vi "RGB_merge.vi"(7 "offset and range":T1[](array[typedef]) {"offset" min=0.0 max=1.0 step=0.0010000000474974513 scale=0.0..1.0; "range" min=0.0 max=1.0 step=0.0010000000474974513 scale=0.0..1.0}, 8 "error in (no error)":errorcluster, 9 "colours":T2[](array[typedef]), 10 "images":refnum<class "Image.lvclass">[](array[class]), 11 "Image in":refnum<class "Image.lvclass">=refnum) -> (0 "error out":errorcluster, 3 "Image out":refnum<class "Image.lvclass">)   [LabVIEW 2010, in "Image.lvclass"]
uses:
  Image.lvclass
  colour_enum.ctl
  clusters/range_offset_cluster.ctl
  storage_mode.ctl
  ErrorController/ErrorController/class_data.vi
  <vilib>/vision/NI_Vision_Development_Module.lvlib
  ErrorController/ErrorController/ErrorController.lvclass
panel:
  # "Note: \nIf offset and range value is not provided or empty, the intrinsic range offset of each image is taken."
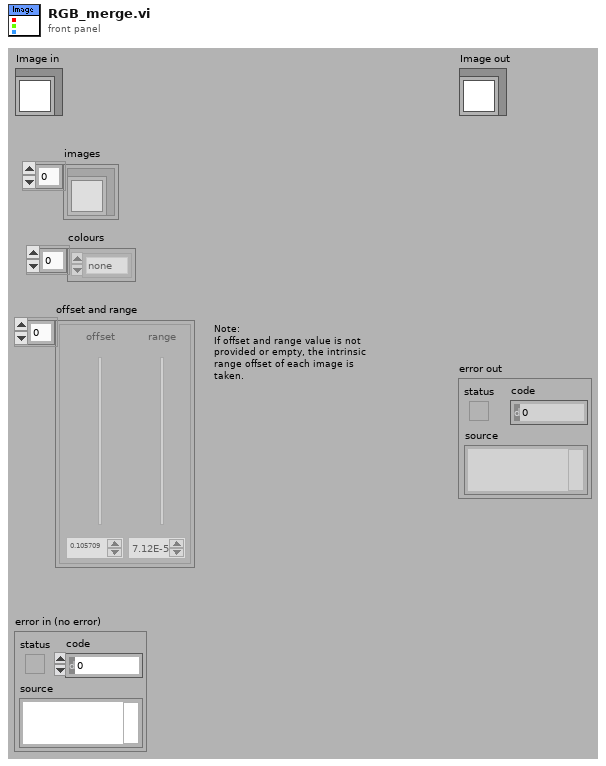
[diagram p1: front panel]
types:
  T1 = typedef "range_offset_cluster.ctl" = cluster{"range":dbl, "offset":dbl}
  T2 = typedef "Image.lvclass/colour_enum.ctl" = enum16{"none", "red", "green", "blue", "grey scale", "custom"}
  T3 = typedef "Image.lvclass/storage_mode.ctl" = enum16{"RAM", "disk"}
  T4 = enum32{"Average", "Min", "Max", "Clear  if < ", "Clear  if < or =", "Clear  if =", "Clear  if > or =", "Clear  if >"}
  T5 = typedef "Image Type" = u32
  T6 = typedef "IMAQ Image.ctl" = refnum<image>
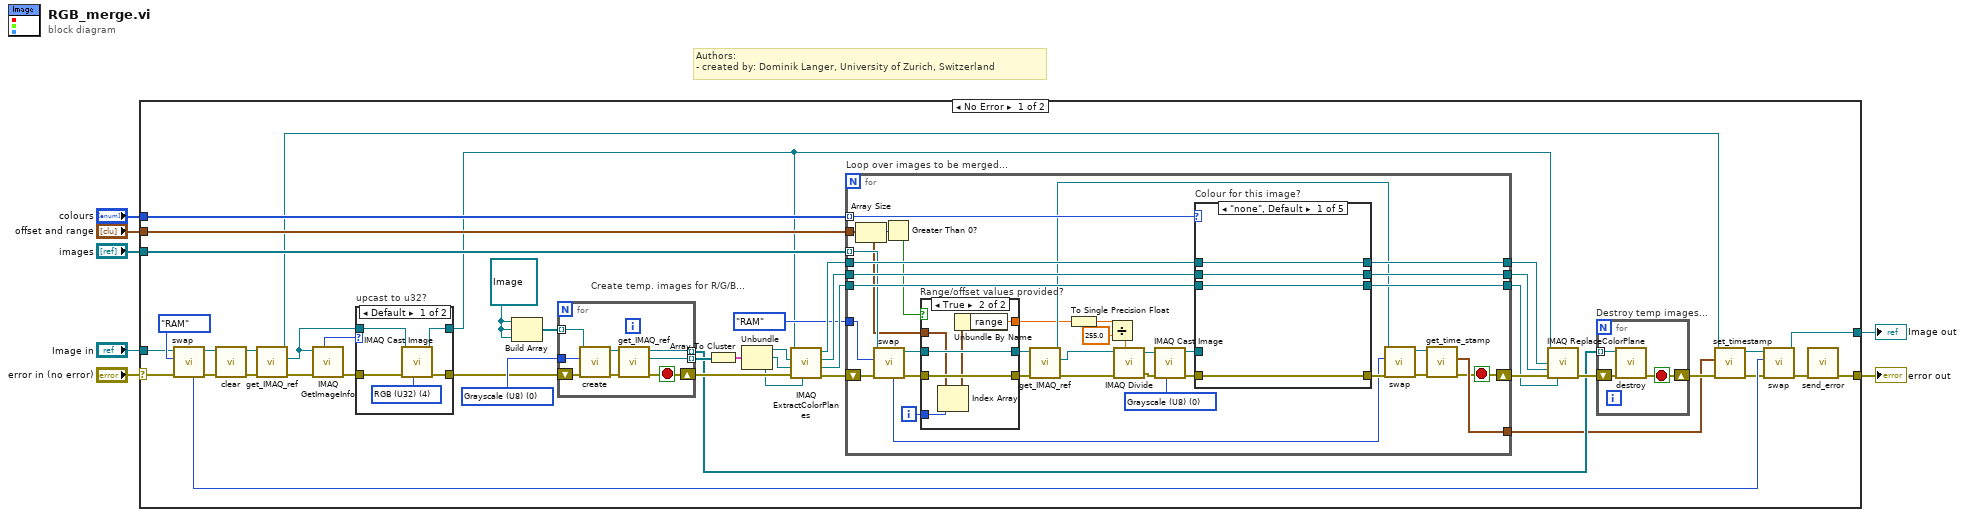
[diagram p0: block diagram]
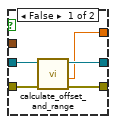
[diagram p3: hidden frame]
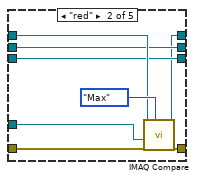
[diagram p4: hidden frame]
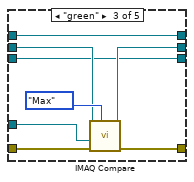
[diagram p5: hidden frame]
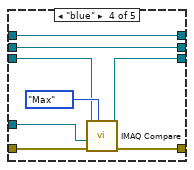
[diagram p6: hidden frame]
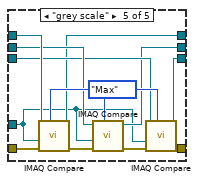
[diagram p7: hidden frame]
diagram:
  # "Authors: \n- created by: Dominik Langer, University of Zurich, Switzerland"
  n1 = case shown="No Error" "error in (no error)" {
    selector: "error in (no error)" -> [w40 w159]
    tunnel: [w8 w159] -> w6
    tunnel: [w37 w158] -> w4
    tunnel: "Image in" -> [w35 w158]
    tunnel: "colours" -> [w48 _]
    tunnel: "images" -> [w47 _]
    tunnel: "offset and range" -> [w22 _]
    frame No Error {
      w29 = refnum<class "Image.lvclass"> refnum ("Image.lvclass")
      w28 = T5 0 items=["Grayscale (U8)", "Grayscale (I16)", "Grayscale (SGL)", "Complex (CSG)", "RGB (U32)", "HSL (U32)", "RGB (U64)"] ("Image Type")
      n2 = call-dynamic "swap.vi"("error in (no error)"=w40, "storage type target"=storage_mode."RAM", "Image in"=w35) -> ("error out"=w39:errorcluster, "Image out"=w38:refnum<class "Image.lvclass">, "previous storage mode"=w34:T3)  [unwired: 6 out]
      n3 = call-dynamic "clear.vi"("error in (no error)"=w39, "Image in"=w38) -> ("error out"=w41:errorcluster, "Image out"=w42:refnum<class "Image.lvclass">)  [unwired: 8 out]
      n4 = call-dynamic "get_IMAQ_ref.vi"("error in (no error)"=w41, "Image.lvclass in"=w42) -> ("error out"=w16:errorcluster, "Image"=w12:T6, "Image.lvclass out"=w19:refnum<class "Image.lvclass">)  [unwired: 7 out]
      n5 = call "IMAQ GetImageInfo"("error in (no error)"=w16, "Image"=w12) -> ("error out"=w13:errorcluster, "Image Type"=w15:T5)  [unwired: 2 in, 6 out]
      n6 = case "upcast to u32?" shown="Default" w15 {
        tunnel: [w53 w59] -> w14
        tunnel: w13 -> [w54 w59]
        tunnel: w12 -> [w57 w58]
        tunnel: [w56 w58] -> w11
        frame Default {
          w55 = T5 4 items=["Grayscale (U8)", "Grayscale (I16)", "Grayscale (SGL)", "Complex (CSG)", "RGB (U32)", "HSL (U32)", "RGB (U64)", "Grayscale (U16)"] ("Image Type")
          n7 = call "IMAQ Cast Image"("Image Type"=w55, "error in (no error)"=w54, "Image Src"=w57) -> ("error out"=w53:errorcluster, "Image Dst Out"=w56:T6)  [unwired: 7 in]
        }
        frame 4 {
        }
      }
      n8 = Build Array(w29, w29, w29) -> (w30:refnum<class "Image.lvclass">[])
      n9 = for "Create temp. images for R/G/B..." {
        shift-right: [w63] -> w27
        shift-left: w14 -> [w68]
        tunnel: [w67] -> w23 mode=indexing
        tunnel: w28 -> [w66]
        tunnel: w30 -> [w65] mode=indexing
        tunnel: [w64] -> w32 mode=indexing
        stop <- w63 stop-if-true
        n10 = call "create.vi"("error in (no error)"=w68, "Image Type"=w66, "Image in"=w65) -> ("error out"=w70:errorcluster, "Image out"=w69:refnum<class "Image.lvclass">)  [unwired: 1 in, 6 out]
        n11 = call-dynamic "get_IMAQ_ref.vi"("error in (no error)"=w70, "Image.lvclass in"=w69) -> ("error out"=w63:errorcluster, "Image"=w64:T6, "Image.lvclass out"=w67:refnum<class "Image.lvclass">)  [unwired: 7 out]
      }
      n12 = Array To Cluster(array=w32) -> (cluster=w31:cluster{"[0]":T6, "[1]":T6, "[2]":T6})
      n13 = Unbundle(w31) -> ("[0]"=w26:T6, "[1]"=w25:T6, "[2]"=w24:T6)
      n14 = call "IMAQ ExtractColorPlanes"("Blue or Luma or Val or Inten Plane"=w24, "error in (no error)"=w27, "Green or Sat Plane"=w25, "Red or Hue Plane"=w26, "Image Src"=w11) -> ("error out"=w10:errorcluster, "Blue or Luma or Val or Inten Plane out"=w44:T6, "Green or Sat Plane out"=w45:T6, "Red or Hue Plane out"=w46:T6)  [unwired: 1 in, 2 out]
      n15 = for "Loop over images to be merged..." {
        tunnel: w48 -> [w106] mode=indexing
        tunnel: w46 -> [w105]
        tunnel: w45 -> [w104]
        tunnel: w44 -> [w103]
        tunnel: [w102] -> w51
        tunnel: [w101] -> w50
        tunnel: [w100] -> w49
        tunnel: w47 -> [w96] mode=indexing
        tunnel: storage_mode."RAM" ("storage type target") -> [w95]
        tunnel: w22 -> [w79]
        tunnel: [w73] -> w17
        shift-right: [w72] -> w52
        shift-left: w10 -> [w71]
        i -> [w78]
        stop <- w72 stop-if-true
        w97 = T5 0 items=["Grayscale (U8)", "Grayscale (I16)", "Grayscale (SGL)", "Complex (CSG)", "RGB (U32)", "HSL (U32)", "RGB (U64)"] ("Image Type")
        n16 = Array Size(array=w79) -> (size(s)=w81:i32)
        n17 = call-dynamic "swap.vi"("error in (no error)"=w71, "storage type target"=w95, "Image in"=w96) -> ("error out"=w91:errorcluster, "Image out"=w90:refnum<class "Image.lvclass">, "previous storage mode"=w92:T3)  [unwired: 6 out]
        n18 = Greater Than 0?(x=w81) -> (x > 0?=w80:bool)
        n19 = case "Range/offset values provided?" shown="True" w80 {
          tunnel: w91 -> [w111 w117]
          tunnel: w90 -> [w110 w116]
          tunnel: [w109 w117] -> w89
          tunnel: [w108 w116] -> w88
          tunnel: [w107 w112] -> w85
          tunnel: w79 -> [_ w115]
          tunnel: w78 -> [_ w114]
          frame False {
            n20 = call-dynamic "calculate_offset_and_range.vi"("error in (no error)"=w111, "Image in"=w110) -> ("error out"=w109:errorcluster, "range"=w107:dbl, "Image out"=w108:refnum<class "Image.lvclass">)  [unwired: 7 out]
          }
          frame True {
            n21 = Index Array(array=w115, index=w114) -> (element=w113:T1)
            n22 = Unbundle By Name(w113) -> ("range"=w112:dbl)
          }
        }
        n23 = call-dynamic "get_IMAQ_ref.vi"("error in (no error)"=w89, "Image.lvclass in"=w88) -> ("error out"=w77:errorcluster, "Image"=w76:T6, "Image.lvclass out"=w93:refnum<class "Image.lvclass">)  [unwired: 7 out]
        n24 = To Single Precision Float(number=w85) -> (single precision float=w84:sgl)
        n25 = Divide(x=w84, y=sgl 255.0) -> (x/y=w82:sgl)
        n26 = call "IMAQ Divide"("Image Src A"=w76, "Constant"=w82, "error in (no error)"=w77) -> ("Image Dst Out"=w86:T6, "error out"=w87:errorcluster)  [unwired: 3 in, 1 out]
        n27 = call "IMAQ Cast Image"("Image Type"=w97, "error in (no error)"=w87, "Image Src"=w86) -> ("error out"=w99:errorcluster, "Image Dst Out"=w98:T6)  [unwired: 3 in, 4 out]
        n28 = case "Colour for this image?" shown="\"none\", Default" w106 {
          tunnel: w105 -> [w121 w126 w132 w139 w156]
          tunnel: w104 -> [w120 w125 w134 w140 w151]
          tunnel: w103 -> [w119 w124 w131 w142 w150]
          tunnel: w99 -> [w118 w128 w135 w143 w157]
          tunnel: [w121 w123 w132 w139 w147] -> w102
          tunnel: [w120 w125 w133 w140 w148] -> w101
          tunnel: [w119 w124 w131 w141 w149] -> w100
          tunnel: [w118 w127 w136 w144 w153] -> w94
          tunnel: w98 -> [_ w122 w130 w138 w146]
          frame "none", Default {
          }
          frame "red" {
            n29 = call "IMAQ Compare"("Operator"=T4."Max", "error in (no error)"=w128, "Image Src B"=w122, "Image Src A"=w126) -> ("error out"=w127:errorcluster, "Image Dst Out"=w123:T6)  [unwired: 2 in, 4 out]
          }
          frame "green" {
            n30 = call "IMAQ Compare"("Operator"=T4."Max", "error in (no error)"=w135, "Image Src B"=w130, "Image Src A"=w134) -> ("error out"=w136:errorcluster, "Image Dst Out"=w133:T6)  [unwired: 2 in, 4 out]
          }
          frame "blue" {
            n31 = call "IMAQ Compare"("Operator"=T4."Max", "error in (no error)"=w143, "Image Src B"=w138, "Image Src A"=w142) -> ("error out"=w144:errorcluster, "Image Dst Out"=w141:T6)  [unwired: 2 in, 4 out]
          }
          frame "grey scale" {
            w152 = T4."Max" ("Operator")
            n32 = call "IMAQ Compare"("Operator"=w152, "error in (no error)"=w157, "Image Src B"=w146, "Image Src A"=w156) -> ("error out"=w155:errorcluster, "Image Dst Out"=w147:T6)  [unwired: 2 in, 4 out]
            n33 = call "IMAQ Compare"("Operator"=w152, "error in (no error)"=w155, "Image Src B"=w146, "Image Src A"=w151) -> ("error out"=w154:errorcluster, "Image Dst Out"=w148:T6)  [unwired: 2 in, 4 out]
            n34 = call "IMAQ Compare"("Operator"=w152, "error in (no error)"=w154, "Image Src B"=w146, "Image Src A"=w150) -> ("error out"=w153:errorcluster, "Image Dst Out"=w149:T6)  [unwired: 2 in, 4 out]
          }
        }
        n35 = call-dynamic "swap.vi"("error in (no error)"=w94, "storage type target"=w92, "Image in"=w93) -> ("error out"=w75:errorcluster, "Image out"=w74:refnum<class "Image.lvclass">)  [unwired: 7 out]
        n36 = call-dynamic "get_time_stamp.vi"("error in (no error)"=w75, "Image.lvclass in"=w74) -> ("error out"=w72:errorcluster, "timestamp"=w73:timestamp)  [unwired: 7 in, 1 out]
      }
      n37 = call "IMAQ ReplaceColorPlane"("Image Src"=w11, "Red or Hue Plane"=w51, "Green or Sat Plane"=w50, "error in (no error)"=w52, "Blue or Luma or Val or Inten Plane"=w49) -> ("error out"=w43:errorcluster)  [unwired: 2 in, 8 out]
      n38 = for "Destroy temp images..." {
        shift-right: [w60] -> w21
        shift-left: w43 -> [w62]
        tunnel: w23 -> [w61] mode=indexing
        stop <- w60 stop-if-true
        n39 = call-dynamic "destroy.vi"("error in (no error)"=w62, "Image in"=w61) -> ("error out"=w60:errorcluster)  [unwired: 9 out]
      }
      n40 = call-dynamic "set_timestamp.vi"("error in (no error)"=w21, "timestamp"=w17, "Image.lvclass in"=w19) -> ("error out"=w20:errorcluster, "Image.lvclass out"=w18:refnum<class "Image.lvclass">)  [unwired: 7 in]
      n41 = call-dynamic "swap.vi"("error in (no error)"=w20, "storage type target"=w34, "Image in"=w18) -> ("error out"=w9:errorcluster, "Image out"=w37:refnum<class "Image.lvclass">)  [unwired: 7 out]
      n42 = call "send_error.vi"("error in (no error)"=w9) -> ("error out"=w8:errorcluster)  [unwired: 10 in]
    }
    frame Error {
    }
  }
  "error out" <- w6
  "Image out" <- w4
